vi "Actor Core.vi"(8 "error in":errorcluster, 11 "Nested in":refnum<class "Kitchen Actor.lvclass">) -> (0 "error out":errorcluster, 3 "Actor out":refnum<class "Actor.lvclass">)   [LabVIEW 2024, in "Kitchen Actor.lvlib" / "Kitchen Actor.lvclass"]
doc: "(<B>Filename</B>: Actor Framework.lvlib:Actor.lvclass:Actor Core.vi)\n\nReceives messages to the actor, reacts to them, and initiates any error handling that may shut the actor down.\n\nDescendant classes may override this VI to append parallel tasks for the actor to complete while it handles messages. Overrides use the Call Parent Method node."
uses:
  Kitchen Actor.lvclass
  C:/Program Files/National Instruments/LabVIEW 2024/vi.lib/ActorFramework/Actor/Actor.lvclass
  <vilib>/ActorFramework/Actor/Actor.lvclass
  <vilib>/Utility/miscctls.llb/LVRectTypeDef.ctl
  <vilib>/ActorFramework/Actor/Actor.lvclass/Actor.ctl
  <vilib>/ActorFramework/Message Enqueuer/Message Enqueuer.lvclass/Message Enqueuer.ctl
  Kitchen Actor.lvclass/Kitchen Actor.ctl
  <vilib>/numeric/Random Number (Range) U64.vi
  <vilib>/ActorFramework/Message Enqueuer/Init from Existing Queue.vi
  <vilib>/ActorFramework/Message Enqueuer/Enqueue.vi
  <vilib>/numeric/sub_Random U32.vi
  <vilib>/ActorFramework/Stop Msg/Stop Msg.lvclass
  C:/Program Files/National Instruments/LabVIEW 2024/vi.lib/ActorFramework/Message/Message.lvclass
  <vilib>/ActorFramework/Message Priority Queue/Priority Enqueue.vi
  <vilib>/ActorFramework/Message Enqueuer/Message Enqueuer.lvclass
panel:
  out "Timer Indicator":string
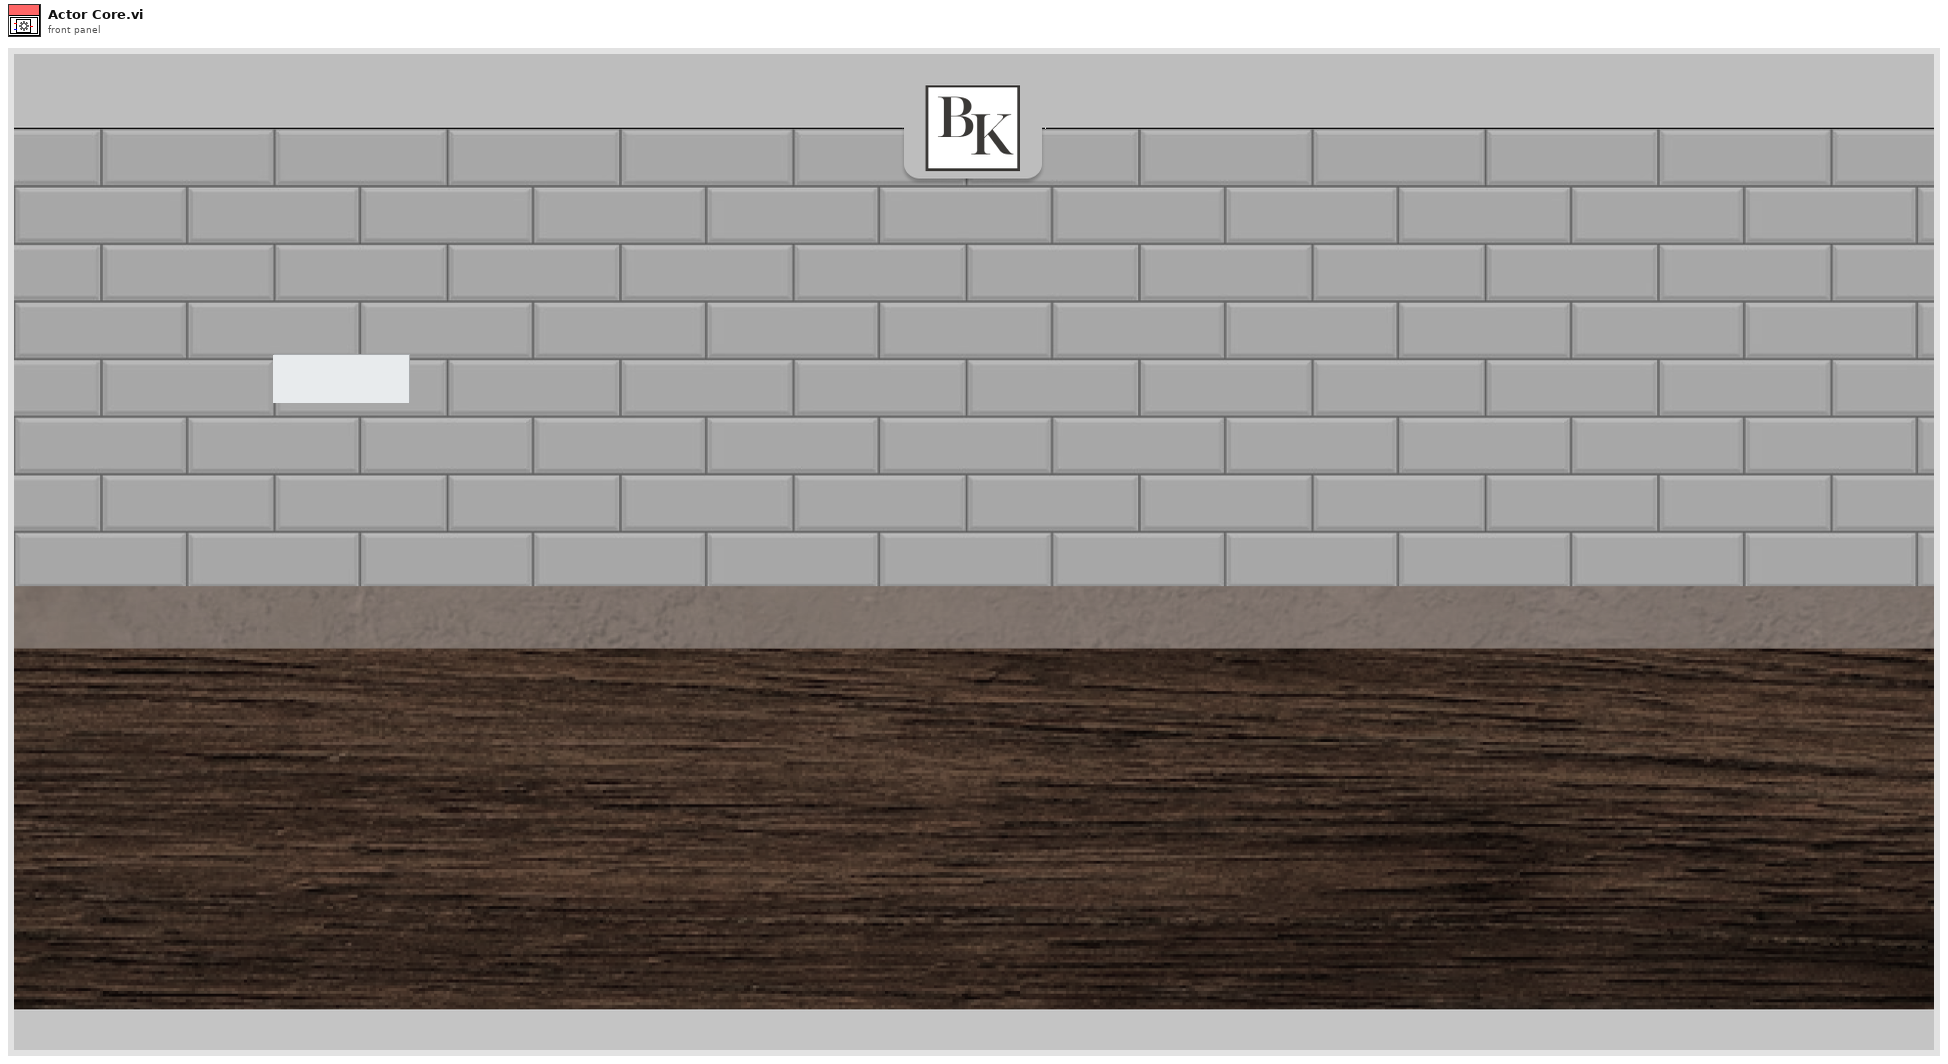
[diagram p1: front panel]
types:
  T1 = typedef "LVRectTypeDef.ctl" = cluster{"Left":i16, "Top":i16, "Right":i16, "Bottom":i16}
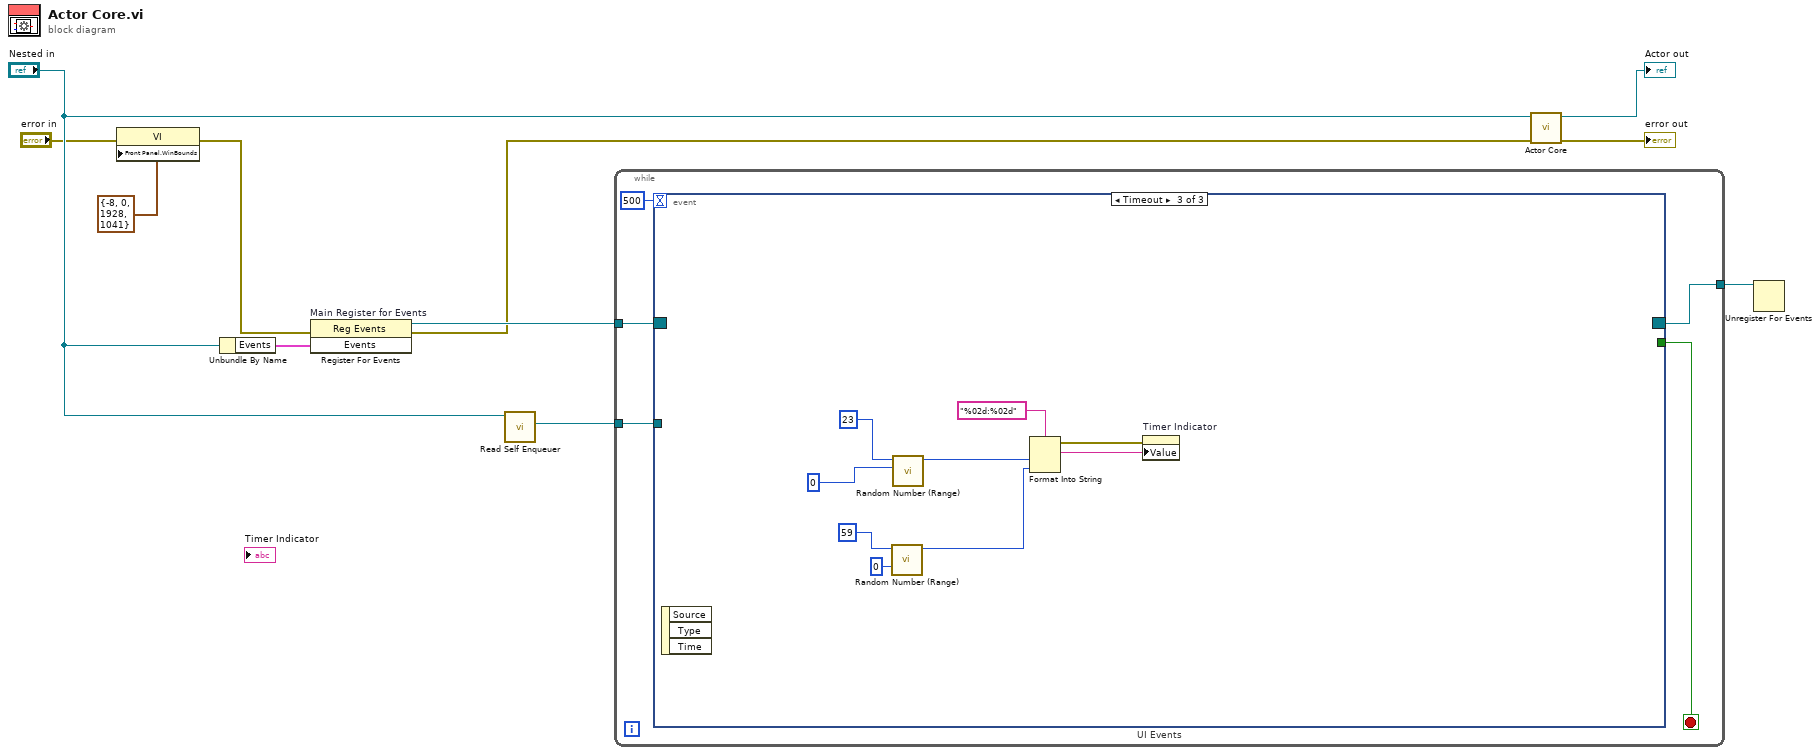
[diagram p0: block diagram]
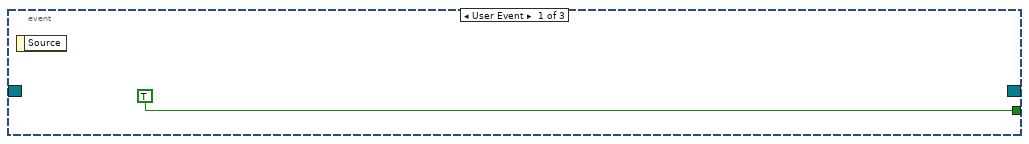
[diagram p2: hidden frame]
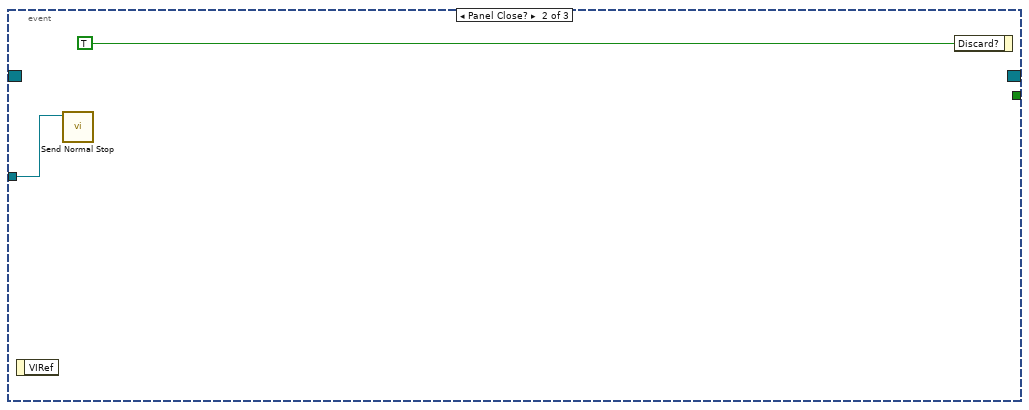
[diagram p3: hidden frame]
diagram:
  n1 = property class="VI"(error in="error in", "Front Panel.WinBounds"=T1 {"Left"=-8, "Top"=0, "Right"=1928, "Bottom"=1041} ("Front Panel Window:Panel Bounds")) -> (error out=w2:errorcluster)  [unwired: 1 in, 1 out]
  n2 = Unbundle By Name("Nested in") -> ("Events"=w8:cluster{"Stop":refnum<user-event>})
  n3 = register-events "Main Register for Events"(error in=w2, w8) -> (reference out=w9:refnum<event-registration>, error out=w4:errorcluster)  [unwired: 1 in]
  n4 = call <vilib>:"Read Self Enqueuer.vi"("Actor"="Nested in") -> ("Self Enqueuer"=w5:refnum<class "Message Enqueuer.lvclass">)  [unwired: 10 in]
  n5 = while {
    tunnel: w9 -> [w16]
    tunnel: [w14] -> w7
    tunnel: w5 -> [w13]
    stop <- w15 stop-if-true
    n6 = event "UI Events" shown="[2] Timeout" {
      selector: w16 -> [_ _ _]
      dyn-events: [_ _ _] -> w14
      timeout: 500 -> [_ _ _]
      tunnel: [TRUE _ _] -> w15
      tunnel: w13 -> [_ w18 _]
      event User Event {
        n7 = event-data() -> ()  [unwired: 1 in, 1 out]
      }
      event Panel Close? {
        n8 = event-data() -> ()  [unwired: 1 in, 1 out]
        n9 = call <vilib>:"Send Normal Stop.vi"("Message Enqueuer"=w18) -> ()  [unwired: 10 in, 1 out]
        n10 = event-data("Discard?"=TRUE) -> ()  [unwired: 1 in, 1 out]
      }
      event Timeout {
        n11 = event-data() -> ()  [unwired: 1 in, 3 out]
        n12 = call-poly <vilib>:"Random Number (Range).vi"("lower bound (0)"=u64 0, "upper bound (100)"=u64 59) -> ("number"=w22:u64)  [unwired: 9 in]
        n13 = call-poly <vilib>:"Random Number (Range).vi"("lower bound (0)"=u64 0, "upper bound (100)"=u64 23) -> ("number"=w26:u64)  [unwired: 9 in]
        n14 = Format Into String(format string="%02d:%02d", w26, w22) -> (resulting string=w27:string, error out=w25:errorcluster)  [unwired: 2 in]
        n15 = property on="Timer Indicator" class="Str"(error in=w25, "Value"=w27) -> ()  [unwired: 1 in, 2 out]
      }
    }
  }
  n16 = call-parent "Actor Core.vi"("error in"=w4, "Actor in"="Nested in") -> ("error out"=→"error out":errorcluster, "Actor out"=→"Actor out":refnum<class "Actor.lvclass">)  [unwired: 8 in]
  n17 = Unregister For Events(event registration refnum=w7) -> ()  [unwired: 1 in, 1 out]
